vi "EnterPosicion2019.vi"(6 "error in (no error)":errorcluster, 8 "ESTADO in":T1) -> (0 "error out":errorcluster, 1 "ESTADO out":T1, 2 "Text":string, 3 "Cancelled?":bool)   [LabVIEW 2013]
doc: "Use this template to create a dialog box. This template polls the state of the buttons on the front panel and does not use events. Use the Dialog Using Events template (not available in Base package) to create a dialog box with event handling."
uses:
  Controles/P2018 Arduino Control.ctl
panel:
  out "Boolean Text.Text":string
  in  "Valvula":bool=TRUE
  in  "Cancel":bool
  in  "OK":bool
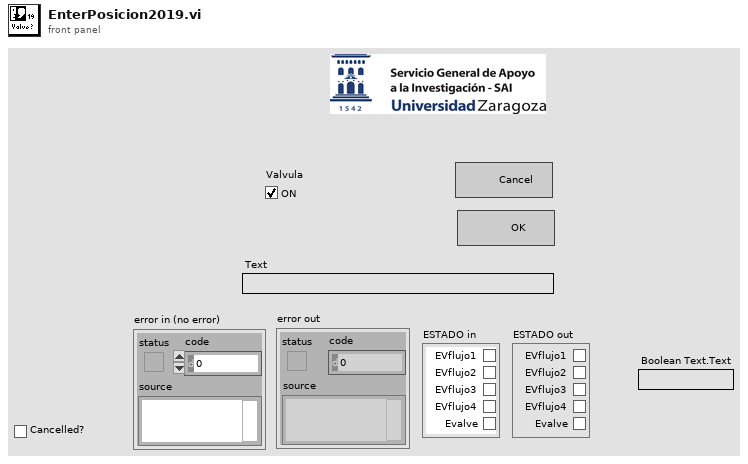
[diagram p1: front panel]
types:
  T1 = typedef "P2018 Arduino Control.ctl" = cluster{"EVflujo1":bool, "EVflujo2":bool, "EVflujo3":bool, "EVflujo4":bool, "Evalve":bool}
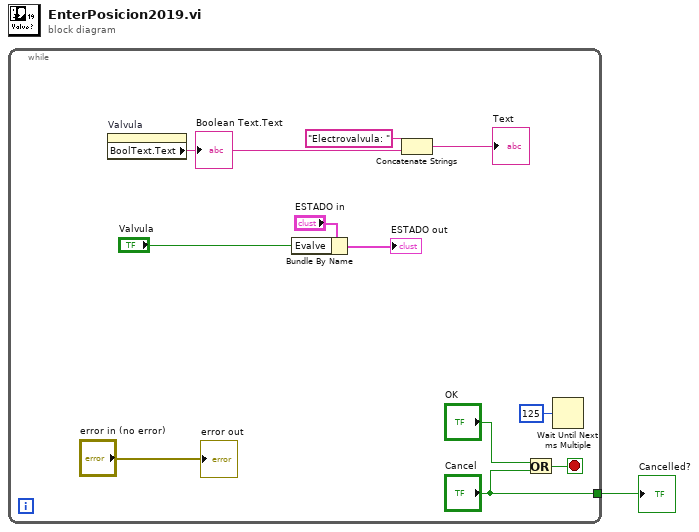
[diagram p0: block diagram]
diagram:
  n1 = while {
    tunnel: ["Cancel"] -> w1
    stop <- w11 stop-if-true
    n2 = property on="Valvula" class="Bool (strict)"() -> ("BoolText.Text"=w7:string)  [unwired: 2 in, 2 out]
    "Boolean Text.Text" <- w7
    n3 = Bundle By Name(cluster="ESTADO in", "Evalve"="Valvula") -> (→"ESTADO out":T1)
    n4 = Concatenate Strings("Electrovalvula: " ("string"), w7) -> (→"Text":string)
    n5 = Or(x="OK", y="Cancel") -> (x .or. y?=w11:bool)
    n6 = Wait Until Next ms Multiple(millisecond multiple=u32 125) -> ()  [unwired: 1 out]
    "error out" <- "error in (no error)"
  }
  "Cancelled?" <- w1
